vi "Spark MAX Process Parameter Stream.vi"(8 "error in (no error)":errorcluster, 11 "SPARK MAX Device Ref in":T1) -> (0 "error out":errorcluster, 3 "SPARK MAX Device Ref out":T1)   [LabVIEW 2023]
uses:
  Typedef/Spark MAX Parameter Status.ctl
  Typedef/Spark MAX Parameter Type.ctl
  Typedef/Spark MAX Parameter Cache Element.ctl
  Typedef/Spark MAX Variant Data.ctl
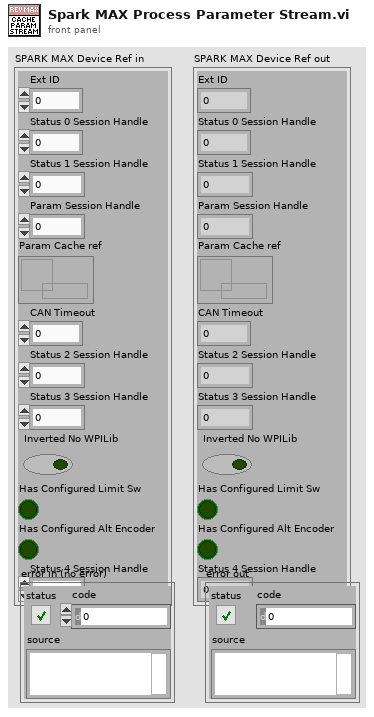
[diagram p1: front panel]
types:
  T1 = typedef "Spark MAX Variant Data.ctl" = cluster{"Ext ID":u32, "Status 0 Session Handle":u32, "Status 1 Session Handle":u32, "Param Session Handle":u32, "Param Cache ref":refnum<data-value>, "CAN Timeout":u32, "Status 2 Session Handle":u32, "Status 3 Session Handle":u32, "Inverted No WPILib":bool, "Has Configured Limit Sw":bool, "Has Configured Alt Encoder":bool, "Status 4 Session Handle":u32}
  T2 = cluster{"Message ID":u32, "Timestamp":u32, "Data":u8[]}[]
  T3 = typedef "Spark MAX Parameter Cache Element.ctl" = cluster{"Timestamp":u32, "Parameter Raw":u32, "Parameter Type":T4, "Last Access Status":T5}
  T4 = typedef "Spark MAX Parameter Type.ctl" = enum16{"Signed Int", "Unsigned Int", "Float", "Bool"}
  T5 = typedef "Spark MAX Parameter Status.ctl" = enum16{"Ok", "Invalid Parameter ID", "Mismatch Type", "Access Mode", "Invalid Parameter Value", "Not Implemented/Depcrecated"}
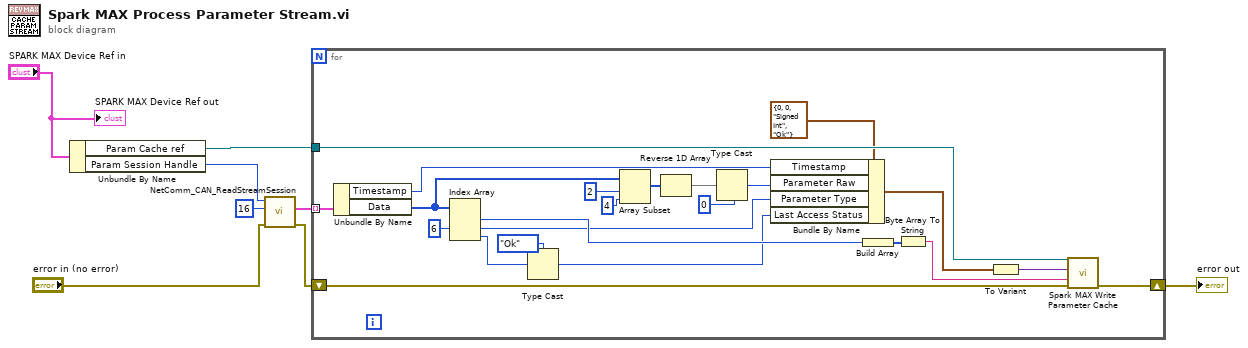
[diagram p0: block diagram]
diagram:
  n1 = Unbundle By Name("SPARK MAX Device Ref in") -> ("Param Cache ref"=w3:refnum<data-value>, "Param Session Handle"=w7:u32)
  n2 = call <vilib>:"NetComm_CAN_ReadStreamSession.vi"("error in (no error)"="error in (no error)", "Messages To Read"=u32 16, "Session Handle"=w7) -> ("error out"=w1:errorcluster, "Messages"=w8:T2)  [unwired: 6 in, 1 out]
  n3 = for {
    shift-right: [w30] -> w4
    shift-left: w1 -> [w31]
    tunnel: w8 -> [w29] mode=indexing
    tunnel: w3 -> [w27]
    n4 = Unbundle By Name(w29) -> ("Timestamp"=w24:u32, "Data"=w21:u8[])
    n5 = Index Array(array=w21, index #2=6 ("index")) -> (element #1=w26:u8, element #2=w22:u8, element #3=w23:u8)  [unwired: 2 in]
    n6 = Type Cast(type=Spark_MAX_Parameter_Status."Ok" ("Parameter Status"), x=w23) -> (*(type *) &x=w9:T5)
    n7 = Array Subset(array=w21, index=2, length=4) -> (w17:u8[])
    n8 = Reverse 1D Array(array=w17) -> (reversed array=w16:u8[])
    n9 = Type Cast(type=u32 0 ("index"), x=w16) -> (*(type *) &x=w14:u32)
    n10 = Bundle By Name(cluster=T3 {"Timestamp"=0, "Parameter Raw"=0, "Parameter Type"=enum."Signed Int", "Last Access Status"=enum."Ok"}, "Timestamp"=w24, "Parameter Raw"=w14, "Parameter Type"=w22, "Last Access Status"=w9) -> (w11:T3)
    n11 = Build Array(w26) -> (w12:u8[])
    n12 = Byte Array To String(unsigned byte array=w12) -> (string=w13:string)
    n13 = To Variant(anything=w11) -> (Variant=w10:variant)
    n14 = call "Spark MAX Write Parameter Cache.vi"("error in (no error)"=w31, "string"=w13, "Variant"=w10, "Data Value Reference in"=w27) -> ("error out"=w30:errorcluster)  [unwired: 7 in]
  }
  "error out" <- w4
  "SPARK MAX Device Ref out" <- "SPARK MAX Device Ref in"
